vi "Variable Instr.vi"() -> ()   [LabVIEW 2020, in "Library Instrument & Equipement.lvlib" / "Library Popup.lvlib" / "Popup Autotest_Without_Actor.lvclass"]
uses:
  Popup Autotest_Without_Actor.lvclass
  Instrument/Instrument (Default)/Class Instrument (Default).lvclass
panel:
  in  "Tableau":T1(array[cluster])
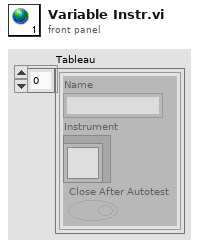
[diagram p1: front panel]
types:
  T1 = cluster{"Name":string, "Instrument":refnum<class "Class Instrument (Default).lvclass">, "Close After Autotest":bool}[]
diagram:
